vi "TOML to Tree.vi"(8 "Tag":string, 9 "Name":string, 10 "Value":T1, 11 "TreeControl in":refnum<vi>) -> (0 "error out":errorcluster)   [LabVIEW 2020]
uses:
  lib/TOML Value.ctl
  lib/TOML Key-Value Pair.ctl
  lib/TOML.lvlib
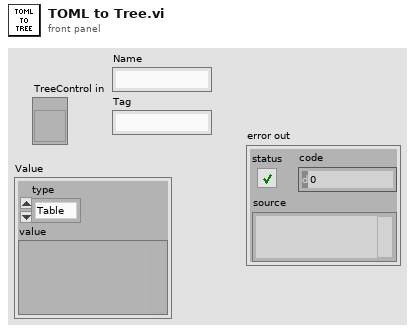
[diagram p1: front panel]
types:
  T1 = typedef "TOML.lvlib/TOML Value.ctl" = cluster{"type":enum16{"Table", "Array", "String", "Integer", "Float", "Boolean", "Offset Date-Time", "Local Date-Time", "Local Date", "Local Time", "Path"}, "value":variant}
  T2 = enum16{"Table", "Array", "String", "Integer", "Float", "Boolean", "Offset Date-Time", "Local Date-Time", "Local Date", "Local Time", "Path"}
  T3 = typedef "TOML.lvlib/TOML Key-Value Pair.ctl" = cluster{"Key":string, "Value":T1}
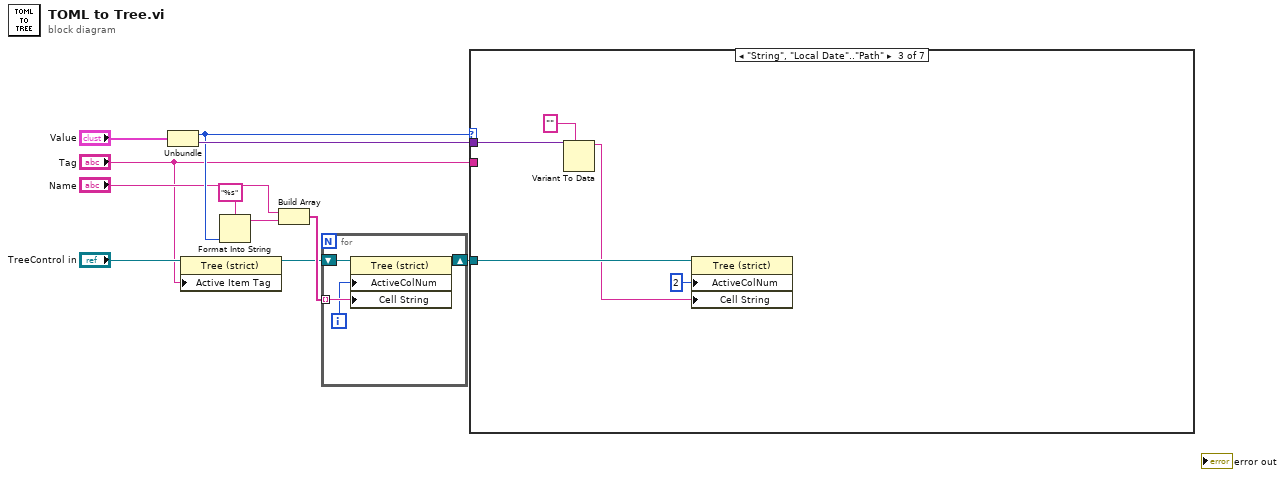
[diagram p0: block diagram]
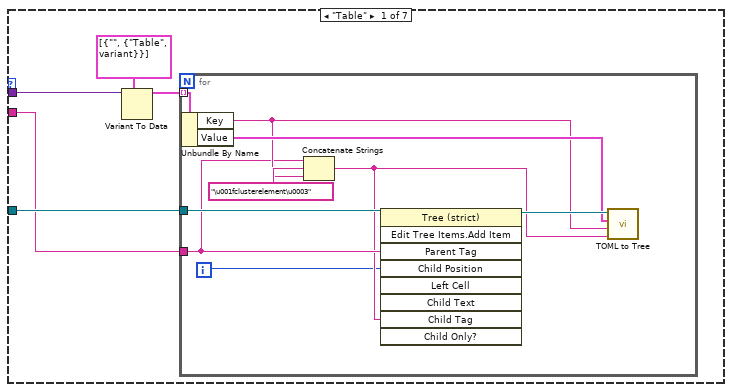
[diagram p2: hidden frame]
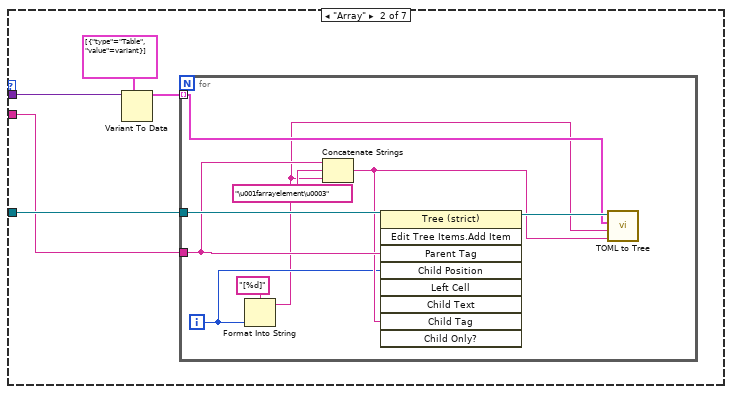
[diagram p3: hidden frame]
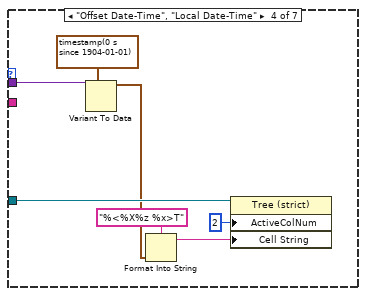
[diagram p4: hidden frame]
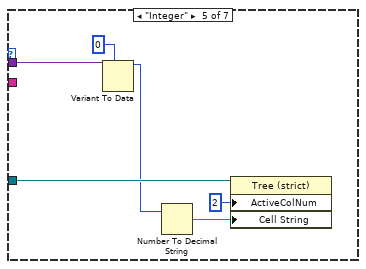
[diagram p5: hidden frame]
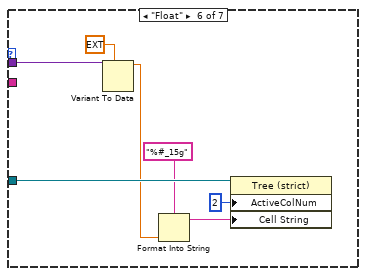
[diagram p6: hidden frame]
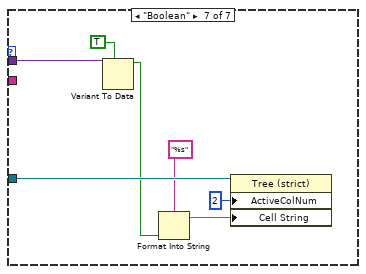
[diagram p7: hidden frame]
diagram:
  n1 = Unbundle("Value") -> ("type"=w8:T2, "value"=w10:variant)
  n2 = property class="Tree (strict)"(reference="TreeControl in", "Active Item Tag"="Tag") -> (reference out=w2:refnum<vi>)  [unwired: 1 in, 1 out]
  n3 = Format Into String(format string="%s", w8) -> (resulting string=w6:string)  [unwired: 2 in, 1 out]
  n4 = Build Array("Name", w6) -> (w5:string[])
  n5 = for {
    tunnel: w5 -> [w14] mode=indexing
    shift-right: [w12] -> w4
    shift-left: w2 -> [w15]
    i -> [w13]
    n6 = property class="Tree (strict)"(reference=w15, "ActiveColNum"=w13, "Cell String"=w14) -> (reference out=w12:refnum<vi>)  [unwired: 1 in, 1 out]
  }
  n7 = case shown="\"String\", \"Local Date\"..\"Path\"" w8 {
    tunnel: w10 -> [w20 w34 w48 w55 w61 w68 w75]
    tunnel: w4 -> [w17 w31 w46 w54 w60 w67 w74]
    tunnel: "Tag" -> [w16 w30 _ _ _ _ _]
    frame "Table" {
      n8 = Variant To Data(type=T3[] [{"Key"="", "Value"={"type"=enum."Table", "value"=variant}}], Variant=w20) -> (data=w18:T3[])  [unwired: 1 in, 1 out]
      n9 = for {
        tunnel: w18 -> [w28] mode=indexing
        tunnel: w16 -> [w23]
        tunnel: w17 -> [w29]
        i -> [w21]
        n10 = Unbundle By Name(w28) -> ("Key"=w24:string, "Value"=w26:T1)
        n11 = Concatenate Strings(w23, "\u001fclusterelement\u0003" ("string"), w24) -> (w22:string)
        n12 = invoke class="Tree (strict)" method="Edit Tree Items.Add Item"(reference=w29, "Parent Tag"=w23, "Child Position"=w21, "Child Tag"=w22) -> (reference out=w27:refnum<vi>)  [unwired: 5 in, 8 out]
        n13 = call "TOML to Tree.vi"("Tag"=w22, "Name"=w24, "Value"=w26, "TreeControl in"=w27) -> ()  [unwired: 7 in, 1 out]
      }
    }
    frame "Array" {
      n14 = Variant To Data(type=T1[] [{"type"=enum."Table", "value"=variant}], Variant=w34) -> (data=w32:T1[])  [unwired: 1 in, 1 out]
      n15 = for {
        tunnel: w32 -> [w38] mode=indexing
        tunnel: w30 -> [w40]
        tunnel: w31 -> [w43]
        i -> [w37]
        n16 = Format Into String(format string="[%d]", w37) -> (resulting string=w35:string)  [unwired: 2 in, 1 out]
        n17 = Concatenate Strings(w40, "\u001farrayelement\u0003" ("string"), w35) -> (w39:string)
        n18 = invoke class="Tree (strict)" method="Edit Tree Items.Add Item"(reference=w43, "Parent Tag"=w40, "Child Position"=w37, "Child Tag"=w39) -> (reference out=w42:refnum<vi>)  [unwired: 5 in, 8 out]
        n19 = call "TOML to Tree.vi"("Tag"=w39, "Name"=w35, "Value"=w38, "TreeControl in"=w42) -> ()  [unwired: 7 in, 1 out]
      }
    }
    frame "String", "Local Date".."Path" {
      n20 = Variant To Data(type="", Variant=w48) -> (data=w44:string)  [unwired: 1 in, 1 out]
      n21 = property class="Tree (strict)"(reference=w46, "ActiveColNum"=2 ("Active Cell:Active Column Number"), "Cell String"=w44) -> ()  [unwired: 1 in, 2 out]
    }
    frame "Offset Date-Time", "Local Date-Time" {
      n22 = Variant To Data(type=timestamp(0 s since 1904-01-01), Variant=w55) -> (data=w51:timestamp)  [unwired: 1 in, 1 out]
      n23 = Format Into String(format string="%<%X%z %x>T", w51) -> (resulting string=w50:string)  [unwired: 2 in, 1 out]
      n24 = property class="Tree (strict)"(reference=w54, "ActiveColNum"=2 ("Active Cell:Active Column Number"), "Cell String"=w50) -> ()  [unwired: 1 in, 2 out]
    }
    frame "Integer" {
      n25 = Variant To Data(type=i64 0, Variant=w61) -> (data=w58:i64)  [unwired: 1 in, 1 out]
      n26 = Number To Decimal String(number=w58) -> (decimal integer string=w56:string)  [unwired: 1 in]
      n27 = property class="Tree (strict)"(reference=w60, "ActiveColNum"=2 ("Active Cell:Active Column Number"), "Cell String"=w56) -> ()  [unwired: 1 in, 2 out]
    }
    frame "Float" {
      n28 = Variant To Data(type=ext 0.0, Variant=w68) -> (data=w64:ext)  [unwired: 1 in, 1 out]
      n29 = Format Into String(format string="%#_15g", w64) -> (resulting string=w63:string)  [unwired: 2 in, 1 out]
      n30 = property class="Tree (strict)"(reference=w67, "ActiveColNum"=2 ("Active Cell:Active Column Number"), "Cell String"=w63) -> ()  [unwired: 1 in, 2 out]
    }
    frame "Boolean" {
      n31 = Variant To Data(type=TRUE, Variant=w75) -> (data=w71:bool)  [unwired: 1 in, 1 out]
      n32 = Format Into String(format string="%s", w71) -> (resulting string=w70:string)  [unwired: 2 in, 1 out]
      n33 = property class="Tree (strict)"(reference=w74, "ActiveColNum"=2 ("Active Cell:Active Column Number"), "Cell String"=w70) -> ()  [unwired: 1 in, 2 out]
    }
  }
